vi "FindHydSens.vi"(3 "booster amp?":bool=TRUE, 4 "Frequency (MHz)":dbl format="%.2f", 5 "Hydrophone":T1) -> (2 "Sensitivity in Pa/V":dbl format="%.2f")   [LabVIEW 2022 SP3]
uses:
  Hydros.ctl
panel:
  out "transposed array":i32[][](array[numeric])
  # "`"
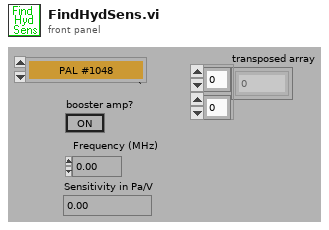
[diagram p1: front panel]
types:
  T1 = typedef "Hydros.ctl" = enum16{"PAL #1048", "PAL #525", "PAL #430a", "PAL #192", "DEAD PAL # 1403", "LOST UHI Onda", "DEAD PAL #1818", "PAL #1974", "DEAD #2266 w/booster", "PAL #2524 w/booster", "PAL FP21-20T", "PAL FP160-13  ", "PAL FP141-20", "PAL FP158-08T"}
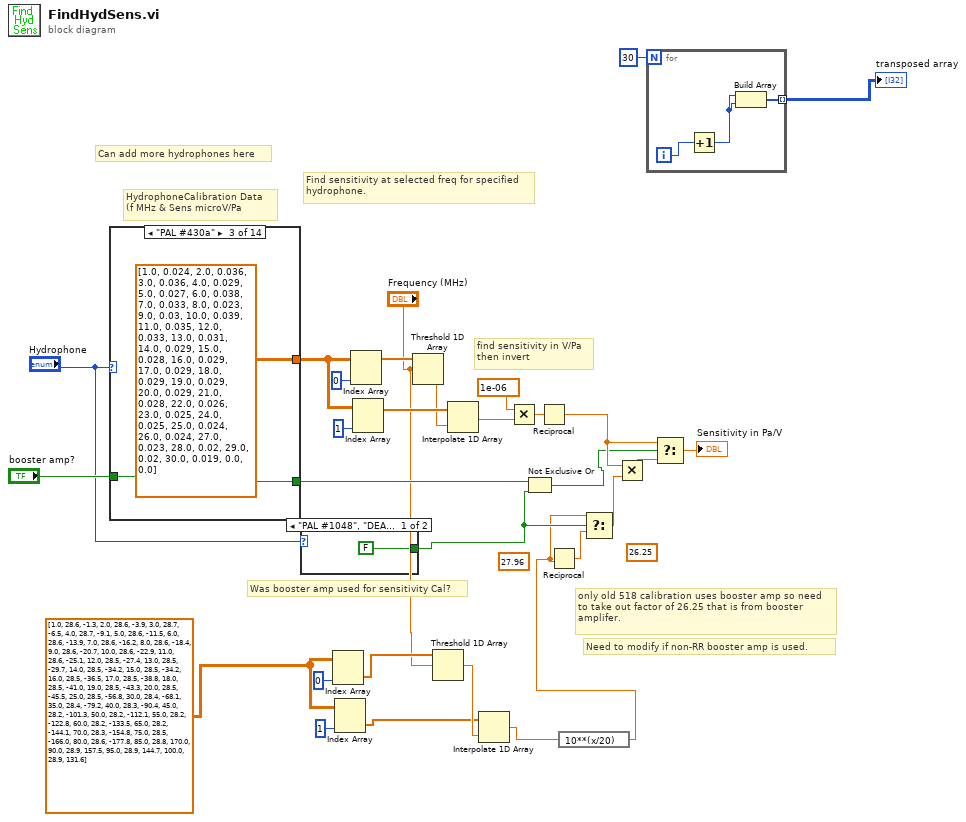
[diagram p0: block diagram]
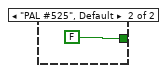
[diagram p2: hidden frame]
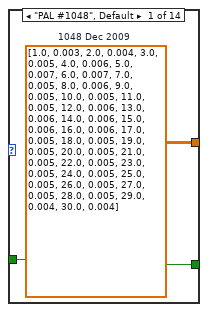
[diagram p3: hidden frame]
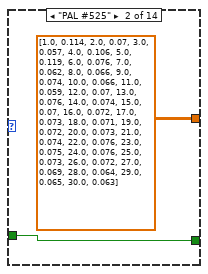
[diagram p4: hidden frame]
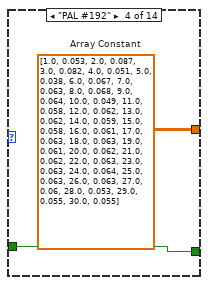
[diagram p5: hidden frame]
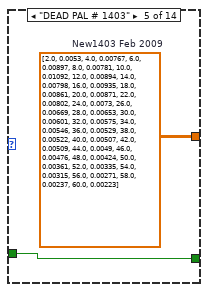
[diagram p6: hidden frame]
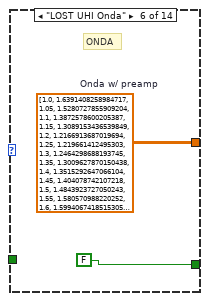
[diagram p7: hidden frame]
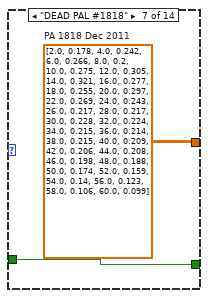
[diagram p8: hidden frame]
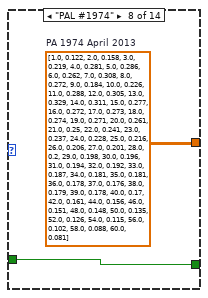
[diagram p9: hidden frame]
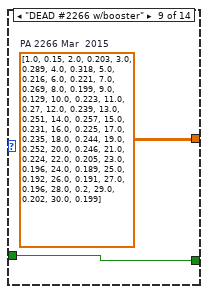
[diagram p10: hidden frame]
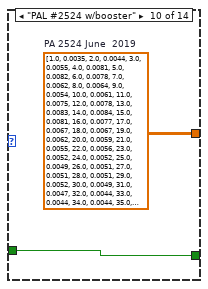
[diagram p11: hidden frame]
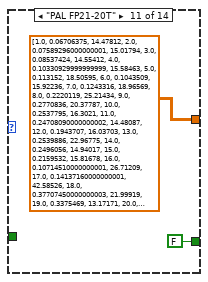
[diagram p12: hidden frame]
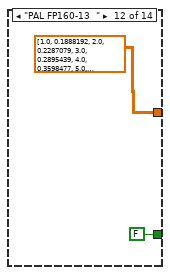
[diagram p13: hidden frame]
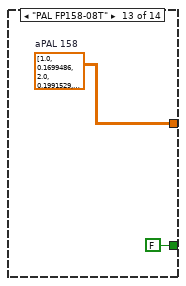
[diagram p14: hidden frame]
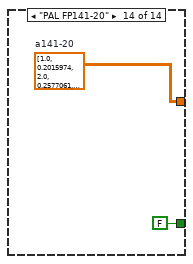
[diagram p15: hidden frame]
diagram:
  w7 = dbl[][] [[1.0, 28.6, -1.3], [2.0, 28.6, -3.9], [3.0, 28.7, -6.5], [4.0, 28.7, -9.1], [5.0, 28.6, -11.5], [6.0, 28.6, -13.9], [7.0, 28.6, -16.2], [8.0, 28.6, -18.4], [9.0, 28.6, -20.7], [10.0, 28.6, -22.9], [11.0, 28.6, -25.1], [12.0, 28.5, -27.4], [13.0, 28.5, -29.7], [14.0, 28.5, -34.2], [15.0, 28.5, -34.2], [16.0, 28.5, -36.5], [17.0, 28.5, -38.8], [18.0, 28.5, -41.0], [19.0, 28.5, -43.3], [20.0, 28.5, -45.5], [25.0, 28.5, -56.8], [30.0, 28.4, -68.1], [35.0, 28.4, -79.2], [40.0, 28.3, -90.4], [45.0, 28.2, -101.3], [50.0, 28.2, -112.1], [55.0, 28.2, -122.8], [60.0, 28.2, -133.5], [65.0, 28.2, -144.1], [70.0, 28.3, -154.8], [75.0, 28.5, -166.0], [80.0, 28.6, -177.8], [85.0, 28.8, 170.0], [90.0, 28.9, 157.5], [95.0, 28.9, 144.7], [100.0, 28.9, 131.6]] ("HydrophoneCalibration Data\n(f MHz & Sens microV/Pa")
  (unwired) 26.25
  (unwired) 27.96
  # "Need to modify if non-RR booster amp is used."
  # "Was booster amp used for sensitivity Cal?"
  # "only old 518 calibration uses booster amp so need to take out factor of 26.25 that is from booster amplifer."
  # "Can add more hydrophones here"
  # "HydrophoneCalibration Data\n(f MHz & Sens microV/Pa"
  # "Find sensitivity at selected freq for specified\nhydrophone."
  # "find sensitivity in V/Pa\nthen invert"
  n1 = case shown="\"PAL #430a\"" "Hydrophone" {
    tunnel: [w32 dbl[][] [[1.0, 0.114], [2.0, 0.07], [3.0, 0.057], [4.0, 0.106], [5.0, 0.119], [6.0, 0.076], [7.0, 0.062], [8.0, 0.066], [9.0, 0.074], [10.0, 0.066], [11.0, 0.059], [12.0, 0.07], [13.0, 0.076], [14.0, 0.074], [15.0, 0.07], [16.0, 0.072], [17.0, 0.073], [18.0, 0.071], [19.0, 0.072], [20.0, 0.073], [21.0, 0.074], [22.0, 0.076], [23.0, 0.075], [24.0, 0.076], [25.0, 0.073], [26.0, 0.072], [27.0, 0.069], [28.0, 0.064], [29.0, 0.065], [30.0, 0.063]] ("HydrophoneCalibration Data\n(f MHz & Sens microV/Pa") dbl[][] [[1.0, 0.024], [2.0, 0.036], [3.0, 0.036], [4.0, 0.029], [5.0, 0.027], [6.0, 0.038], [7.0, 0.033], [8.0, 0.023], [9.0, 0.03], [10.0, 0.039], [11.0, 0.035], [12.0, 0.033], [13.0, 0.031], [14.0, 0.029], [15.0, 0.028], [16.0, 0.029], [17.0, 0.029], [18.0, 0.029], [19.0, 0.029], [20.0, 0.029], [21.0, 0.028], [22.0, 0.026], [23.0, 0.025], [24.0, 0.025], [25.0, 0.024], [26.0, 0.024], [27.0, 0.023], [28.0, 0.02], [29.0, 0.02], [30.0, 0.019], [0.0, 0.0]] ("HydrophoneCalibration Data\n(f MHz & Sens microV/Pa") w38 w40 w41 w43 w45 w47 w49 dbl[][] [[1.0, 0.06706375, 14.47812], [2.0, 0.07589296000000001, 15.01794], [3.0, 0.08537424, 14.55412], [4.0, 0.10330929999999999, 15.58463], [5.0, 0.113152, 18.50595], [6.0, 0.1043509, 15.92236], [7.0, 0.1243316, 18.96569], [8.0, 0.2220119, 25.21434], [9.0, 0.2770836, 20.37787], [10.0, 0.2537795, 16.3021], [11.0, 0.24708090000000002, 14.48087], [12.0, 0.1943707, 16.03703], [13.0, 0.2539886, 22.96775], [14.0, 0.2496056, 14.94017], [15.0, 0.2159532, 15.81678], [16.0, 0.10714510000000001, 26.71209], [17.0, 0.14137160000000001, 42.58526], [18.0, 0.37707450000000003, 21.99919], [19.0, 0.3375469, 13.17171], [20.0, 0.32497859999999995, 24.38966], [21.0, 0.3366132, 25.92397], [22.0, 0.2035944, 36.81563], [23.0, 0.08916912, 39.03531], [24.0, 0.17409460000000002, 62.63712], [25.0, 0.3071859, 37.05608], [26.0, 0.3782059, 28.066], [27.0, 0.289014, 45.75546], [28.0, 0.28804050000000003, 50.94493], [29.0, 0.27057749999999997, 101.1496], [30.0, 0.2382274, 14.24891], [31.0, 0.235338, 71.46823], [32.0, 0.22686060000000002, 66.79519], [33.0, 0.2649338, 23.98092], [34.0, 0.19701580000000002, 50.31683], [35.0, 0.216312, 44.139], [36.0, 0.29565440000000004, 21.03454], [37.0, 0.32125990000000004, 21.22452], [38.0, 0.2798641, 18.62937], [39.0, 0.26867430000000003, 18.42782], [40.0, 0.2726423, 22.3509]] ("all rows") dbl[][] [[1.0, 0.1888192], [2.0, 0.2287079], [3.0, 0.2895439], [4.0, 0.3598477], [5.0, 0.45229700000000006], [6.0, 0.5354445], [7.0, 0.6017091], [8.0, 0.6444105], [9.0, 0.6811724], [10.0, 0.6572835], [11.0, 0.7612123000000001], [12.0, 0.6316092], [13.0, 0.5381608999999999], [14.0, 0.4961414], [15.0, 0.6593777000000001], [16.0, 0.7856242], [17.0, 0.6276374], [18.0, 0.402186], [19.0, 0.2519606], [20.0, 0.4291704], [21.0, 0.5744374], [22.0, 0.7414599], [23.0, 0.9717657000000001], [24.0, 1.0995519999999999], [25.0, 1.346301], [26.0, 1.180118], [27.0, 0.7183915], [28.0, 0.3827823], [29.0, 0.1987299], [30.0, 0.4426664], [31.0, 0.4511647], [32.0, 0.5610603], [33.0, 0.8053196], [34.0, 0.9409113], [35.0, 0.9166176], [36.0, 0.7597702000000001], [37.0, 0.8266086], [38.0, 0.6275379000000001], [39.0, 0.5141969000000001], [40.0, 0.359077]] ("all rows") w55 w57] -> w22
    tunnel: "booster amp?" -> [w31 w33 w35 w37 w39 _ w44 w46 w48 w50 _ _ _ _]
    tunnel: [w31 w33 w35 w37 w39 FALSE w44 w46 w48 w50 FALSE ("booster amp?") FALSE ("booster amp?") FALSE ("booster amp?") FALSE ("booster amp?")] -> w14
    frame "PAL #1048", Default {
      w32 = dbl[][] [[1.0, 0.003], [2.0, 0.004], [3.0, 0.005], [4.0, 0.006], [5.0, 0.007], [6.0, 0.007], [7.0, 0.005], [8.0, 0.006], [9.0, 0.005], [10.0, 0.005], [11.0, 0.005], [12.0, 0.006], [13.0, 0.006], [14.0, 0.006], [15.0, 0.006], [16.0, 0.006], [17.0, 0.005], [18.0, 0.005], [19.0, 0.005], [20.0, 0.005], [21.0, 0.005], [22.0, 0.005], [23.0, 0.005], [24.0, 0.005], [25.0, 0.005], [26.0, 0.005], [27.0, 0.005], [28.0, 0.005], [29.0, 0.004], [30.0, 0.004]]  # 1048 Dec 2009
    }
    frame "PAL #525" {
    }
    frame "PAL #430a" {
    }
    frame "PAL #192" {
      w38 = dbl[][] [[1.0, 0.053], [2.0, 0.087], [3.0, 0.082], [4.0, 0.051], [5.0, 0.038], [6.0, 0.067], [7.0, 0.063], [8.0, 0.068], [9.0, 0.064], [10.0, 0.049], [11.0, 0.058], [12.0, 0.062], [13.0, 0.062], [14.0, 0.059], [15.0, 0.058], [16.0, 0.061], [17.0, 0.063], [18.0, 0.063], [19.0, 0.061], [20.0, 0.062], [21.0, 0.062], [22.0, 0.063], [23.0, 0.063], [24.0, 0.064], [25.0, 0.063], [26.0, 0.063], [27.0, 0.06], [28.0, 0.053], [29.0, 0.055], [30.0, 0.055]]  # Array Constant
    }
    frame "DEAD PAL # 1403" {
      w40 = dbl[][] [[2.0, 0.0053], [4.0, 0.00767], [6.0, 0.00897], [8.0, 0.00781], [10.0, 0.01092], [12.0, 0.00894], [14.0, 0.00798], [16.0, 0.00935], [18.0, 0.00861], [20.0, 0.00871], [22.0, 0.00802], [24.0, 0.0073], [26.0, 0.00669], [28.0, 0.00653], [30.0, 0.00601], [32.0, 0.00575], [34.0, 0.00546], [36.0, 0.00529], [38.0, 0.00522], [40.0, 0.00507], [42.0, 0.00509], [44.0, 0.0049], [46.0, 0.00476], [48.0, 0.00424], [50.0, 0.00361], [52.0, 0.00335], [54.0, 0.00315], [56.0, 0.00271], [58.0, 0.00237], [60.0, 0.00223]]  # New1403 Feb 2009
    }
    frame "LOST UHI Onda" {
      w41 = dbl[][] [[1.0, 1.6391408258984717], [1.05, 1.5280727855909204], [1.1, 1.3872578600205387], [1.15, 1.3089153436539849], [1.2, 1.2166913687019694], [1.25, 1.219661412495303], [1.3, 1.2464298688193745], [1.35, 1.3009627870150438], [1.4, 1.3515292647066104], [1.45, 1.404078742107218], [1.5, 1.4843923727050243], [1.55, 1.580570988220252], [1.6, 1.5994067418515305], [1.65, 1.6658379697122967], [1.7, 1.7302860211000393], [1.75, 1.7481305560103393], [1.8, 1.7451523963595583], [1.85, 1.8214995830686151], [1.9, 1.8452940332517513], [1.95, 1.9047848439408537], [2.0, 1.473454684504832], [2.05, 1.3861960275952498], [2.1, 1.4635359511213772], [2.15, 1.5220364390571053], [2.2, 1.566655272806765], [2.25, 1.5567388766054704], [2.3, 1.5527720056644558], [2.35, 1.523025028695795], [2.4, 1.5914419665484034], [2.45, 1.5874758232420858], [2.5, 1.5696281409781816], [2.55, 1.6003667531228574], [2.6, 1.5944181766690353], [2.65, 1.5825204042090202], [2.7, 1.6192090720768613], [2.75, 1.596404661258997], [2.8, 1.622186755933904], [2.85, 1.6271463283822238], [2.9, 1.6132664971846793], [2.95, 1.5874881100134042], [3.0, 1.5993892666752703], [3.05, 1.635088117357472], [3.1, 1.5815464288372323], [3.15, 1.6063385402973378], [3.2, 1.6112995015746276], [3.25, 1.5875051937427178], [3.3, 1.6063485627326668], [3.35, 1.571647141611164], [3.4, 1.5250467527706353], [3.45, 1.5081937357918664], [3.5, 1.5508357990216466], [3.55, 1.5557980280937251], [3.6, 1.5617519358749168], [3.65, 1.6113361625514406], [3.7, 1.6400973354627217], [3.75, 1.6559680512445387], [3.8, 1.6777886779774904], [3.85, 1.7204332730810643], [3.9, 1.721430777433305], [3.95, 1.7452355550730574], [4.0, 1.7254095967169127], [4.05, 1.7531813870016666], [4.1, 1.7779786613311783], [4.15, 1.711546595997261], [4.2, 1.6520556945073557], [4.25, 1.7185019044713248], [4.3, 1.6957013565758023], [4.35, 1.7690901385877718], [4.4, 1.7512481168279177], [4.45, 1.7621640310382087], [4.5, 1.7730801800430969], [4.55, 1.7681299309749363], [4.6, 1.76218818153291], [4.65, 1.763188197993796], [4.7, 1.7592299163005736], [4.75, 1.8068391107282358], [4.8, 1.7235465654381623], [4.85, 1.7374389009753357], [4.9, 1.7404228046260062], [4.95, 1.7711744427354184], [5.0, 1.785067561962298], [5.05, 1.8822644792540428], [5.1, 1.8128545695570806], [5.15, 1.8614586663549535], [5.2, 1.873369585109904], [5.25, 1.8773469251759578], [5.3, 1.9160351533828814], [5.35, 1.839681857704246], [5.4, 1.8396924163507418], [5.45, 1.8377195273390508], [5.5, 1.8149198000940394], [5.55, 1.8347658444905157], [5.6, 1.7901470531288726], [5.65, 1.8050344874287758], [5.7, 1.7772755517318046], [5.75, 1.7981140079305666], [5.8, 1.781264620997867], [5.85, 1.7981363342624832], [5.9, 1.7703769607016362], [5.95, 1.7654291561333817], [6.0, 1.796186806841966], [6.05, 1.8358714164146601], [6.1, 1.8636546663399967], [6.15, 1.8349034686020949], [6.2, 1.8607035631891722], [6.25, 1.8131069437987934], [6.3, 1.8230376620329358], [6.35, 1.8161068410828605], [6.4, 1.7992572499450217], [6.45, 1.803237021609951], [6.5, 1.834989714732989], [6.55, 1.823099666189795], [6.6, 1.814185202832122], [6.65, 1.780472990664439], [6.7, 1.8142105708768161], [6.75, 1.8142233627982132], [6.8, 1.796381569200965], [6.85, 1.7894508536972995], [6.9, 1.8341010783268161], [6.95, 1.8043558625327354], [7.0, 1.8261920019682802], [7.05, 1.8906829471216118], [7.1, 1.8430822258116317], [7.15, 1.8917027514191207], [7.2, 1.8857648276219705], [7.25, 1.8808189264166317], [7.3, 1.858016987116143], [7.35, 1.8352148199686904], [7.4, 1.8590370105959269], [7.45, 1.8689714237450379], [7.5, 1.8094638189352885], [7.55, 1.8600716560509556], [7.6, 1.8650462042344134], [7.65, 1.888869958678459], [7.7, 1.845233959092183], [7.75, 1.92560594637717], [7.8, 1.8819697054436988], [7.85, 1.8393249026875012], [7.9, 1.8373552573435354], [7.95, 1.875069702602231], [8.0, 1.8750846733761655], [8.05, 1.8701391710027178], [8.1, 1.8890046096185833], [8.15, 1.918783846200127], [8.2, 1.8910195335074782], [8.25, 1.9128622285445092], [8.3, 1.9505798230153826], [8.35, 1.9168622838390916], [8.4, 1.934737287979521], [8.45, 1.9536047354477886], [8.5, 1.922863200937263], [8.55, 1.9228793181786887], [8.6, 1.9139656152576563], [8.65, 1.8802464346886252], [8.7, 1.9397958058657492], [8.75, 1.9447734293600454], [8.8, 1.9120461957017914], [8.85, 1.927938533934011], [8.9, 1.9279552040300434], [8.95, 1.8991961382021347], [9.0, 1.8873053990183606], [9.05, 1.9270131873419676], [9.1, 1.8764231754596776], [9.15, 1.8625475437754206], [9.2, 1.8933255337341712], [9.25, 1.8923500594240164], [9.3, 1.925113700992119], [9.35, 1.9420006537332681], [9.4, 1.924155880591369], [9.45, 1.965852083248996], [9.5, 1.9688470008940486], [9.55, 1.9708496950822763], [9.6, 1.9559819821434976], [9.65, 1.9589771016971158], [9.7, 1.9381547968235802], [9.75, 1.9093929322656855], [9.8, 1.934221149728804], [9.85, 1.91042095462119], [9.9, 1.9729623792509667], [9.95, 1.947177383444212], [10.0, 1.9323089866445335], [10.05, 1.9283574959105962], [10.1, 1.9323458008474013], [10.15, 1.9244244692752255], [10.2, 1.9919324989732425], [10.25, 2.0167643242432662], [10.3, 2.0217465466206215], [10.35, 2.0267288820067044], [10.4, 2.0287338037203337], [10.45, 1.9493505504293307], [10.5, 1.951354909667723], [10.55, 1.8918206865164804], [10.6, 1.9017652925212283], [10.65, 1.9524059739534236], [10.7, 1.9315812899345357], [10.75, 1.8650966267682265], [10.8, 1.8631303811113429], [10.85, 1.830392916051741], [10.9, 1.8383527800293888], [10.95, 1.8731142493539548], [11.0, 1.8880234110242755], [11.05, 1.9257642336081495], [11.1, 1.9168503700446986], [11.15, 1.8721998020057677], [11.2, 1.8642780662242548], [11.25, 1.81069190260986], [11.3, 1.8146820947972917], [11.35, 1.7680434481194451], [11.4, 1.8266339637476179], [11.45, 1.8246682595691481], [11.5, 1.836601227830251], [11.55, 1.8445634372008937], [11.6, 1.8892588189320862], [11.65, 1.8992075838991642], [11.7, 1.8525670693751033], [11.75, 1.8208177494027862], [11.8, 1.8039601742639795], [11.85, 1.7811453138435083], [11.9, 1.7821583377169912], [11.95, 1.7702643927361956], [12.0, 1.7782275894471458], [12.05, 1.796119917575514], [12.1, 1.7455032406439475], [12.15, 1.7504880499626365], [12.2, 1.7802959309134712], [12.25, 1.796203684979216], [12.3, 1.7654438157905668], [12.35, 1.7366692047377328], [12.4, 1.755556203267449], [12.45, 1.8151557054525014], [12.5, 1.660271846903535], [12.55, 1.6682359240937008], [12.6, 1.689109443939587], [12.65, 1.7000533788692909], [12.7, 1.7199350119854946], [12.75, 1.7566989970385642], [12.8, 1.751755552016855], [12.85, 1.698151620134502], [12.9, 1.7011522256532938], [12.95, 1.6922358674463938], [13.0, 1.6624640642101425], [13.05, 1.6366641445305385], [13.1, 1.6436370979467212], [13.15, 1.6744458634159318], [13.2, 1.6814196930802223], [13.25, 1.6854142888697015], [13.3, 1.690402323223011], [13.35, 1.6973769868099424], [13.4, 1.715277266465691], [13.45, 1.6586862681023695], [13.5, 1.5832223190031305], [13.55, 1.552452813337303], [13.6, 1.548500726942839], [13.65, 1.5346158681711433], [13.7, 1.5743685439896469], [13.75, 1.5992227971113788], [13.8, 1.5763985059905772], [13.85, 1.5515870341831075], [13.9, 1.6370365500508726], [13.95, 1.63109932988644], [14.0, 1.60926805316873], [14.05, 1.597370124668497], [14.1, 1.5874588165905485], [14.15, 1.5129752197312891], [14.2, 1.5050494917533062], [14.25, 1.5110319200610645], [14.3, 1.5170146170712007], [14.35, 1.5359127604616443], [14.4, 1.529974342281622], [14.45, 1.5349643891516822], [14.5, 1.531013037909055], [14.55, 1.4614884524099316], [14.6, 1.4436264111992778], [14.65, 1.4386802762297068], [14.7, 1.4476442048008462], [14.75, 1.479461170902294], [14.8, 1.4586179393000673], [14.85, 1.4377741410413643], [14.9, 1.4387899069113115], [14.95, 1.4447740772397626], [15.0, 1.4527458707534664], [15.05, 1.440844293562034], [15.1, 1.4001251329210773], [15.15, 1.4001471750274423], [15.2, 1.416069058573704], [15.25, 1.4339790279223192], [15.3, 1.4081640207758672], [15.35, 1.4061990575253454], [15.4, 1.4092030887354579], [15.45, 1.4092258543563168], [15.5, 1.35856350514416], [15.55, 1.3347333796794154], [15.6, 1.3297859567522283], [15.65, 1.3238445846659175], [15.7, 1.3338053749613867], [15.75, 1.3477422516442419], [15.8, 1.3388193607390764], [15.85, 1.342817547009826], [15.9, 1.3428401063020943], [15.95, 1.3130434374391045], [16.0, 1.2792698879294508], [16.05, 1.2792916211588465], [16.1, 1.3329909640564779], [16.15, 1.3409661592895552], [16.2, 1.3340307675110732], [16.25, 1.3211307809659152], [16.3, 1.2605138221320813], [16.35, 1.234688805014024], [16.4, 1.2834227672591183], [16.45, 1.2923925839741692], [16.5, 1.2924152984459942], [16.55, 1.2954206600400335], [16.6, 1.2437451542255973], [16.65, 1.2069811793033554], [16.7, 1.2149565812939493], [16.75, 1.2219380946747562], [16.8, 1.2279256647246923], [16.85, 1.236896395125425], [16.9, 1.2259813458698732], [16.95, 1.2051227386213434], [17.0, 1.1942068553632805], [17.05, 1.183290660652693], [17.1, 1.1723741272611872], [17.15, 1.175378827669607], [17.2, 1.1674451319644241], [17.25, 1.1436002356946444], [17.3, 1.1585382095571204], [17.35, 1.175465727098014], [17.4, 1.1565922865013776], [17.45, 1.1526358380195936], [17.5, 1.159619103416751], [17.55, 1.1675972333169722], [17.6, 1.1626463531992033], [17.65, 1.1348199347488084], [17.7, 1.142798220715143], [17.75, 1.1527660768016301], [17.8, 1.1378683691968157], [17.85, 1.1408739989758059], [17.9, 1.15581593693846], [17.95, 1.1637956204379563], [18.0, 1.1588443511315143], [18.05, 1.1061456284220699], [18.1, 1.1051721539610344], [18.15, 1.1400105327557637], [18.2, 1.1350586022691074], [18.25, 1.11617913044009], [18.3, 1.083371340139736], [18.35, 1.0804078439212337], [18.4, 1.0993313839450067], [18.45, 1.1033323793605174], [18.5, 1.0963895565611401], [18.55, 1.0645732918846997], [18.6, 1.0576294942434457], [18.65, 1.0904841632843978], [18.7, 1.1074203452007774], [18.75, 1.12037721040078], [18.8, 1.1164191680540236], [18.85, 1.11246100760351], [18.9, 1.1104928242998469], [18.95, 1.1144951210697507], [19.0, 1.1234730969144602], [19.05, 1.1185197307474999], [19.1, 1.1115758887127412], [19.15, 1.102641480448914], [19.2, 1.0956970877472327], [19.25, 1.0957188731790313], [19.3, 1.0927549883247492], [19.35, 1.0848147961596473], [19.4, 1.0788648354924915], [19.45, 1.0729146286979663], [19.5, 1.0629830058857666], [19.55, 1.0620088876415006], [19.6, 1.0928856911139362], [19.65, 1.0968889616412942], [19.7, 1.0590863581786276], [19.75, 1.0431810878796894], [19.8, 1.0422065087418804], [19.85, 1.0472045519752666], [19.9, 1.0551891759127752], [19.95, 1.0621786317084905], [20.0, 1.068172882827096]]  # Onda w/ preamp
      # "ONDA"
    }
    frame "DEAD PAL #1818" {
      w43 = dbl[][] [[2.0, 0.178], [4.0, 0.242], [6.0, 0.266], [8.0, 0.2], [10.0, 0.275], [12.0, 0.305], [14.0, 0.321], [16.0, 0.277], [18.0, 0.255], [20.0, 0.297], [22.0, 0.269], [24.0, 0.243], [26.0, 0.217], [28.0, 0.217], [30.0, 0.228], [32.0, 0.224], [34.0, 0.215], [36.0, 0.214], [38.0, 0.215], [40.0, 0.209], [42.0, 0.206], [44.0, 0.208], [46.0, 0.198], [48.0, 0.188], [50.0, 0.174], [52.0, 0.159], [54.0, 0.14], [56.0, 0.123], [58.0, 0.106], [60.0, 0.099]]  # PA 1818 Dec 2011
    }
    frame "PAL #1974" {
      w45 = dbl[][] [[1.0, 0.122], [2.0, 0.158], [3.0, 0.219], [4.0, 0.281], [5.0, 0.286], [6.0, 0.262], [7.0, 0.308], [8.0, 0.272], [9.0, 0.184], [10.0, 0.226], [11.0, 0.288], [12.0, 0.305], [13.0, 0.329], [14.0, 0.311], [15.0, 0.277], [16.0, 0.272], [17.0, 0.273], [18.0, 0.274], [19.0, 0.271], [20.0, 0.261], [21.0, 0.25], [22.0, 0.241], [23.0, 0.237], [24.0, 0.228], [25.0, 0.216], [26.0, 0.206], [27.0, 0.201], [28.0, 0.2], [29.0, 0.198], [30.0, 0.196], [31.0, 0.194], [32.0, 0.192], [33.0, 0.187], [34.0, 0.181], [35.0, 0.181], [36.0, 0.178], [37.0, 0.176], [38.0, 0.179], [39.0, 0.178], [40.0, 0.17], [42.0, 0.161], [44.0, 0.156], [46.0, 0.151], [48.0, 0.148], [50.0, 0.135], [52.0, 0.126], [54.0, 0.115], [56.0, 0.102], [58.0, 0.088], [60.0, 0.081]]  # PA 1974 April 2013
    }
    frame "DEAD #2266 w/booster" {
      w47 = dbl[][] [[1.0, 0.15], [2.0, 0.203], [3.0, 0.289], [4.0, 0.318], [5.0, 0.216], [6.0, 0.221], [7.0, 0.269], [8.0, 0.199], [9.0, 0.129], [10.0, 0.223], [11.0, 0.27], [12.0, 0.239], [13.0, 0.251], [14.0, 0.257], [15.0, 0.231], [16.0, 0.225], [17.0, 0.235], [18.0, 0.244], [19.0, 0.252], [20.0, 0.246], [21.0, 0.224], [22.0, 0.205], [23.0, 0.196], [24.0, 0.189], [25.0, 0.192], [26.0, 0.191], [27.0, 0.196], [28.0, 0.2], [29.0, 0.202], [30.0, 0.199]]  # PA 2266 Mar  2015
    }
    frame "PAL #2524 w/booster" {
      w49 = dbl[][] [[1.0, 0.0035], [2.0, 0.0044], [3.0, 0.0055], [4.0, 0.0081], [5.0, 0.0082], [6.0, 0.0078], [7.0, 0.0062], [8.0, 0.0064], [9.0, 0.0054], [10.0, 0.0061], [11.0, 0.0075], [12.0, 0.0078], [13.0, 0.0083], [14.0, 0.0084], [15.0, 0.0081], [16.0, 0.0077], [17.0, 0.0067], [18.0, 0.0067], [19.0, 0.0062], [20.0, 0.0059], [21.0, 0.0055], [22.0, 0.0056], [23.0, 0.0052], [24.0, 0.0052], [25.0, 0.0049], [26.0, 0.0051], [27.0, 0.0051], [28.0, 0.0051], [29.0, 0.0052], [30.0, 0.0049], [31.0, 0.0047], [32.0, 0.0044], [33.0, 0.0044], [34.0, 0.0044], [35.0, 0.0044], [36.0, 0.0043], [37.0, 0.0041], [38.0, 0.0038], [39.0, 0.0036], [40.0, 0.0037]]  # PA 2524 June  2019
    }
    frame "PAL FP21-20T" {
    }
    frame "PAL FP160-13  " {
    }
    frame "PAL FP158-08T" {
      w55 = dbl[][] [[1.0, 0.1699486], [2.0, 0.1991529], [3.0, 0.2244326], [4.0, 0.27789569999999997], [5.0, 0.34330309999999997], [6.0, 0.39667610000000003], [7.0, 0.43818070000000003], [8.0, 0.4915227], [9.0, 0.5210666], [10.0, 0.5462136000000001], [11.0, 0.5566911999999999], [12.0, 0.5706136], [13.0, 0.5831534], [14.0, 0.6046401], [15.0, 0.6450766], [16.0, 0.5275818000000001], [17.0, 0.10964109999999999], [18.0, 0.27444510000000005], [19.0, 0.4032876], [20.0, 0.4255527], [21.0, 0.4425725], [22.0, 0.4805593], [23.0, 0.5406155], [24.0, 0.6386779], [25.0, 0.6961022], [26.0, 0.5668044999999999], [27.0, 0.5997295], [28.0, 0.670857], [29.0, 0.6357865], [30.0, 0.5490335000000001], [31.0, 0.5831855], [32.0, 0.5947474], [33.0, 0.7024602], [34.0, 0.7262315], [35.0, 0.744518], [36.0, 0.7601366], [37.0, 0.7653221], [38.0, 0.7272849], [39.0, 0.7429013999999999], [40.0, 0.7399782]]  # aPAL 158
    }
    frame "PAL FP141-20" {
      w57 = dbl[][] [[1.0, 0.2015974], [2.0, 0.2577061], [3.0, 0.33654180000000006], [4.0, 0.4487149], [5.0, 0.6012141000000001], [6.0, 0.6801851000000001], [7.0, 0.7793722000000001], [8.0, 0.803277], [9.0, 0.7860129], [10.0, 0.8016835], [11.0, 0.7577861], [12.0, 0.9032705999999999], [13.0, 0.9614827], [14.0, 0.7313158], [15.0, 0.47134660000000006], [16.0, 0.4717306], [17.0, 0.7226571], [18.0, 1.0345050000000002], [19.0, 1.179571], [20.0, 1.380303], [21.0, 1.273587], [22.0, 0.8011905], [23.0, 0.3254007], [24.0, 0.5309294999999999], [25.0, 1.055142], [26.0, 1.025651], [27.0, 0.5264181], [28.0, 0.2029928], [29.0, 0.7099204], [30.0, 1.074343], [31.0, 1.140363], [32.0, 1.028326], [33.0, 0.64605], [34.0, 0.2514255], [35.0, 0.5067092], [36.0, 0.4019864], [37.0, 0.3400259], [38.0, 0.3208683], [39.0, 0.4513745], [40.0, 0.41702140000000004]]  # a141-20
    }
  }
  n2 = case shown="\"PAL #1048\", \"DEAD PAL #1818\"..\"DEAD #2266 w/booster\"" "Hydrophone" {
    tunnel: [FALSE FALSE] -> w13
    frame "PAL #1048", "DEAD PAL #1818".."DEAD #2266 w/booster" {
    }
    frame "PAL #525", Default {
    }
  }
  n3 = Index Array(array=w7, index (col)=0 ("Index")) -> (element=w6:dbl[])  [unwired: 1 in]
  n4 = Index Array(array=w7, index (col)=1 ("Index")) -> (element=w2:dbl[])  [unwired: 1 in]
  n5 = Index Array(array=w22, index (col)=0 ("Index")) -> (element=w29:dbl[])  [unwired: 1 in]
  n6 = Index Array(array=w22, index (col)=1 ("Index")) -> (element=w28:dbl[])  [unwired: 1 in]
  n7 = Threshold 1D Array(2:"Frequency (MHz)", 3:w29) -> (0:w24:dbl)  [unwired: 1 out]
  n8 = Threshold 1D Array(2:"Frequency (MHz)", 3:w6) -> (0:w3:dbl)  [unwired: 1 out]
  n9 = Interpolate 1D Array(1:w24, 2:w28) -> (0:w27:dbl)
  n10 = Interpolate 1D Array(1:w3, 2:w2) -> (0:w1:dbl)
  n11 = Multiply(x=1e-06, y=w27) -> (x*y=w25:dbl)
  n12 = Not Exclusive Or(1:w13, 2:w14) -> (0:w16:bool)
  n13 = Reciprocal(x=w25) -> (1/x=w20:dbl)
  n14 = expression code="10**(x/20)"(w1) -> (w4:dbl)
  n15 = Reciprocal(x=w4) -> (1/x=w19:dbl)
  n16 = Select(t=w4, s=w13, f=w19) -> (s? t:f=w18:dbl)
  n17 = Multiply(x=w20, y=w18) -> (x*y=w21:dbl)
  n18 = for {
    N: 30 -> [_]
    tunnel: [w61] -> w11 mode=indexing
    i -> [w63]
    n19 = Increment(x=w63) -> (x+1=w62:i32)
    n20 = Build Array(w62, w62) -> (w61:i32[])
  }
  "transposed array" <- w11
  n21 = Select(t=w20, s=w16, f=w21) -> (s? t:f=→"Sensitivity in Pa/V":dbl)
